vi "Append.vi"(8 "error in (no error)":errorcluster, 10 "list node":refnum<class "ListNode.lvclass">, 11 "List in":refnum<class "DoubleLinkedList.lvclass">) -> (0 "error out":errorcluster, 3 "List out":refnum<class "DoubleLinkedList.lvclass">)   [LabVIEW 2010, in "DoubleLinkedList.lvclass"]
uses:
  DoubleLinkedList.lvclass
  ListNode/ListNode.lvclass
  ListNodeVirtual/ListNodeVirtual.lvclass
  DoubleLinkedList.lvclass/DoubleLinkedList.ctl
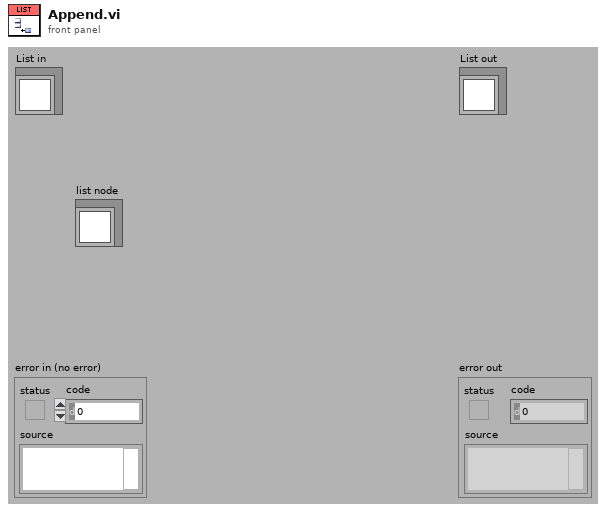
[diagram p1: front panel]
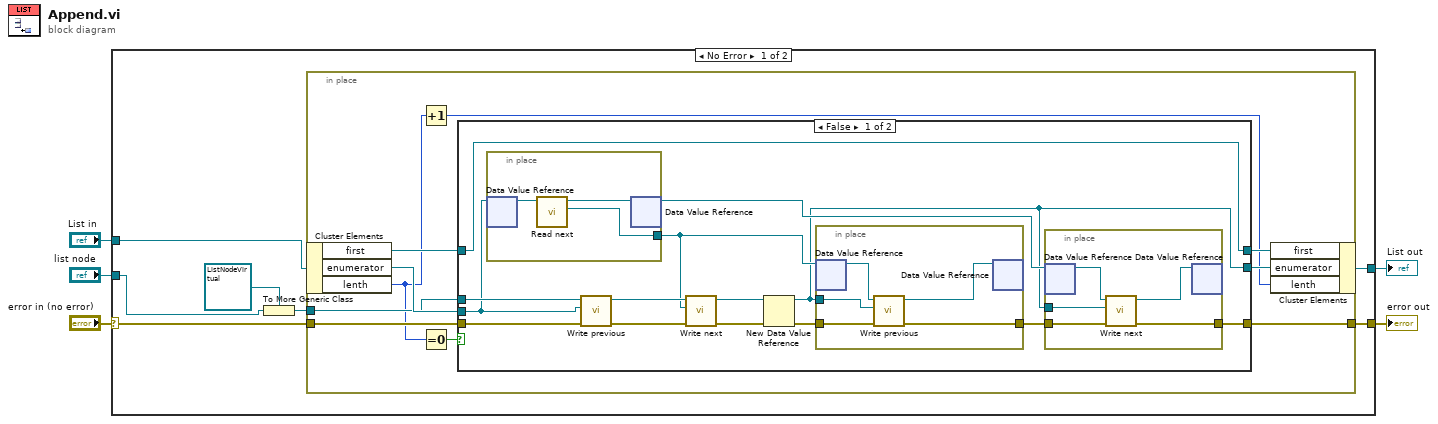
[diagram p0: block diagram]
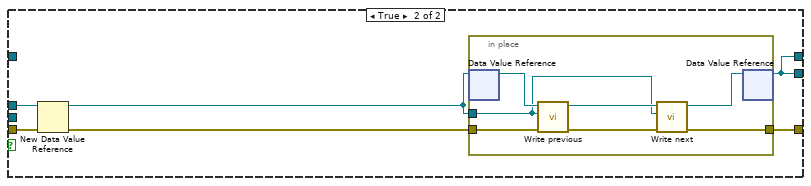
[diagram p2: hidden frame]
diagram:
  n1 = case shown="No Error" "error in (no error)" {
    selector: "error in (no error)" -> [w10 w64]
    tunnel: [w9 w64] -> w4
    tunnel: [w11 w63] -> w2
    tunnel: "List in" -> [w12 w63]
    tunnel: "list node" -> [w8 _]
    frame No Error {
      n2 = To More Generic Class(target class=refnum<class "ListNodeVirtual.lvclass"> refnum ("ListNodeVirtual.lvclass"), reference=w8) -> (generic class reference=w7:refnum<class "ListNodeVirtual.lvclass">)
      n3 = in-place {
        in-place-border: w7 -> [w20]
        in-place-border: w10 -> [w19]
        in-place-border: [w18] -> w9
        n4 = in-place-cluster #1(w12) -> ("first"=w16:refnum<data-value>, "enumerator"=w22:refnum<data-value>, "lenth"=w14:u32)
        n5 = Increment(x=w14) -> (x+1=w13:u32)
        n6 = Equal To 0?(x=w14) -> (x = 0?=w15:bool)
        n7 = case shown="False" w15 {
          tunnel: w22 -> [w33 _]
          tunnel: [w24 w51] -> w21
          tunnel: w20 -> [w36 w50]
          tunnel: w19 -> [w35 w54]
          tunnel: [w26 w52] -> w18
          tunnel: [w34 w51] -> w17
          tunnel: w16 -> [w34 _]
          frame False {
            n8 = in-place {
              in-place-border: [w48] -> w28
              n9 = in-place-dvr #2(w33) -> (w49:refnum<class "ListNodeVirtual.lvclass">)  [unwired: 1 out]
              n10 = call-dynamic "Read next.vi"("NodeType in"=w49) -> ("next"=w48:refnum<data-value>, "NodeType out"=w47:refnum<class "ListNodeVirtual.lvclass">)  [unwired: 8 in, 1 out]
              n11 = in-place-dvr #2(w47) -> (w25:refnum<data-value>)  [unwired: 1 out]
            }
            n12 = call-dynamic "Write previous.vi"("error in (no error)"=w35, "previous"=w33, "NodeType in"=w36) -> ("error out"=w30:errorcluster, "NodeType out"=w29:refnum<class "ListNodeVirtual.lvclass">)  [unwired: 7 in]
            n13 = call-dynamic "Write next.vi"("error in (no error)"=w30, "next"=w28, "NodeType in"=w29) -> ("error out"=w27:errorcluster, "NodeType out"=w23:refnum<class "ListNodeVirtual.lvclass">)  [unwired: 7 in]
            n14 = New Data Value Reference(data value=w23, error in=w27) -> (data value reference=w24:refnum<data-value>, error out=w32:errorcluster)
            n15 = in-place {
              in-place-border: w24 -> [w46]
              in-place-border: w32 -> [w43]
              in-place-border: [w45] -> w31
              n16 = in-place-dvr #3(w28) -> (w44:refnum<class "ListNodeVirtual.lvclass">)  [unwired: 1 out]
              n17 = call-dynamic "Write previous.vi"("error in (no error)"=w43, "previous"=w46, "NodeType in"=w44) -> ("error out"=w45:errorcluster, "NodeType out"=w42:refnum<class "ListNodeVirtual.lvclass">)  [unwired: 7 in]
              n18 = in-place-dvr #3(w42) -> ()  [unwired: 2 out]
            }
            n19 = in-place {
              in-place-border: w24 -> [w41]
              in-place-border: w31 -> [w39]
              in-place-border: [w38] -> w26
              n20 = in-place-dvr #4(w25) -> (w40:refnum<class "ListNodeVirtual.lvclass">)  [unwired: 1 out]
              n21 = call-dynamic "Write next.vi"("error in (no error)"=w39, "next"=w41, "NodeType in"=w40) -> ("error out"=w38:errorcluster, "NodeType out"=w37:refnum<class "ListNodeVirtual.lvclass">)  [unwired: 7 in]
              n22 = in-place-dvr #4(w37) -> ()  [unwired: 2 out]
            }
          }
          frame True {
            n23 = New Data Value Reference(data value=w50, error in=w54) -> (data value reference=w53:refnum<data-value>, error out=w55:errorcluster)
            n24 = in-place {
              in-place-border: w55 -> [w58]
              in-place-border: w53 -> [w57]
              in-place-border: [w60] -> w52
              n25 = in-place-dvr #5(w53) -> (w59:refnum<class "ListNodeVirtual.lvclass">)  [unwired: 1 out]
              n26 = call-dynamic "Write previous.vi"("error in (no error)"=w58, "previous"=w57, "NodeType in"=w59) -> ("error out"=w61:errorcluster, "NodeType out"=w62:refnum<class "ListNodeVirtual.lvclass">)  [unwired: 7 in]
              n27 = call-dynamic "Write next.vi"("error in (no error)"=w61, "next"=w57, "NodeType in"=w62) -> ("error out"=w60:errorcluster, "NodeType out"=w56:refnum<class "ListNodeVirtual.lvclass">)  [unwired: 7 in]
              n28 = in-place-dvr #5(w56) -> (w51:refnum<data-value>)  [unwired: 1 out]
            }
          }
        }
        n29 = in-place-cluster #1("first"=w17, "enumerator"=w21, "lenth"=w13) -> (w11:refnum<class "DoubleLinkedList.lvclass">)
      }
    }
    frame Error {
    }
  }
  "error out" <- w4
  "List out" <- w2
